vi "S8300E_ENT_TEST_MODE_DVT.vi"() -> ()   [LabVIEW 2011]
panel:
  out "Found login?":bool
  out "TELNET-KEYWORD2-AfterLogin":string
  out "TELNET-KEYWORD1-AfterLogin":string
  out "TELNET-PATH":string
  out "TELNET-PASSWORD":string
  out "TELNET-ID":string
  out "Debug View":string
  out "cmd-list":T1(array[cluster])
  out "cmd":string
  out "VISA resource name out":refnum<visa-resource-name>
  out "進行狀況":string
  out "BEGIN TIME":u32
  # "Error Code:MB-NG"
  # "S8300E Enter Test Mode"
  # "2015-1-26"
  # "COM9 115200"
  # "1.本程式不會給UUT 上電,需先執行上電程式\n2.在執行本程式前,需先執行上電程式(S8300E_BootupTime_Delay)\n3.本程式只是給UUT ROOT權限 與 切換到測試程式路徑"
  # "Write Command :Char by Char"
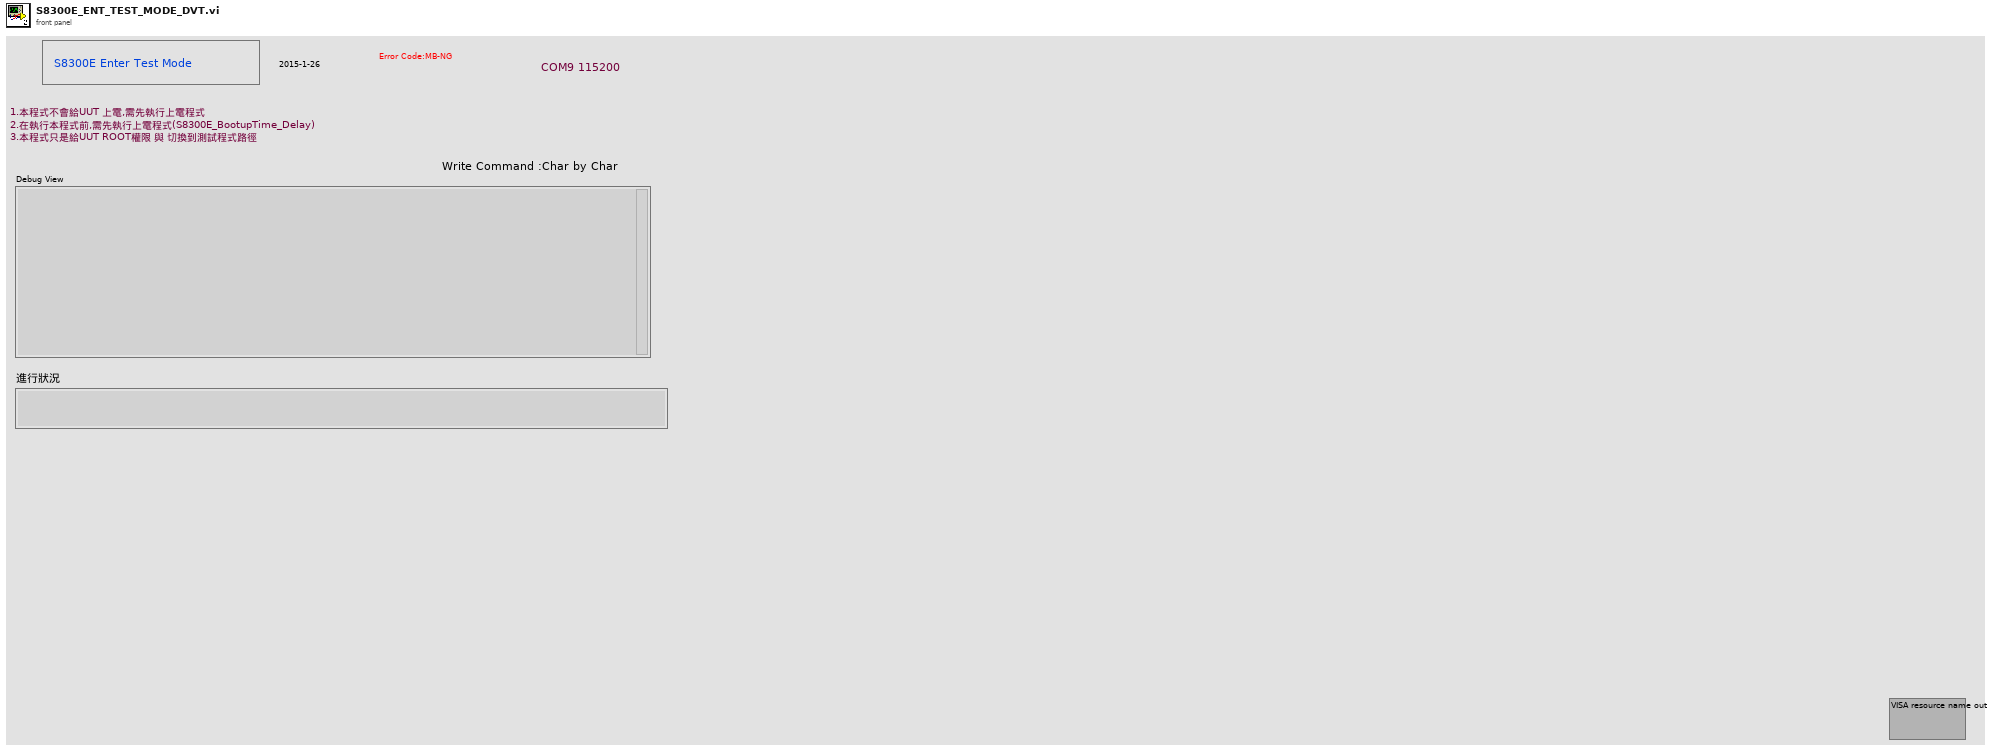
[diagram p1: front panel]
types:
  T1 = cluster{string, "Find this String":string, "Status":string}[]
  T2 = cluster{string, "TELNET-KEYWORD1-AfterLogin":string, "Status":string}
  T3 = cluster{string, "Search String":string, "Status":string}
  T4 = cluster{string, "TELNET-KEYWORD2-AfterLogin":string, "Status":string}
  T5 = cluster{string, "TELNET-KEYWORD2-AfterLogin":string, "Status":string}[]
  T6 = cluster{string, "Find this String":string, "Status":string}
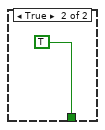
[diagram p4: hidden frame]
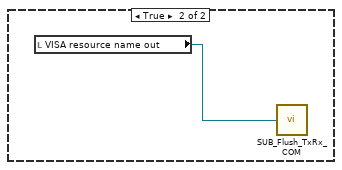
[diagram p5: hidden frame]
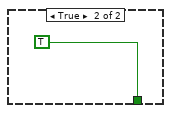
[diagram p7: hidden frame]
diagram:
  n1 = flat-sequence {
    tunnel: [w38] -> w2
    tunnel: w2 -> [w39]
    tunnel: [w144] -> w1
    tunnel: w1 -> [w150]
    frame #0 {
      n2 = Tick Count (ms)() -> (millisecond timer value=→"BEGIN TIME":u32)
    }
    frame #1 {
      n3 = call "SUB_COM1_CLOSE.vi"("VISA resource name"=refnum<visa-resource-name> "COM9") -> ()  [unwired: 3 in]
      n4 = property on="進行狀況" class="Str"("Blinking"=TRUE) -> ()  [unwired: 2 in, 2 out]
      "進行狀況" <- "進入測試準備中...." ("進行狀況")
      "Debug View" <- ""
    }
    frame #2 {
      n5 = call "SUB_COM9_INIT.vi"("baud rate"=u32 115200) -> ("VISA resource name out"=→"VISA resource name out":refnum<visa-resource-name>)  [unwired: 1 in, 1 out]
    }
    frame #3 {
      n6 = call "SUB_ReadScript_File.vi"("Script FileName"="S8300E_sfcs_misc.txt" ("Search Filename in Folder")) -> ("text"=w18:string)  [unwired: 1 in, 2 out]
      n7 = call "SUB_FindSpecificString.vi"("Find this String"="TELNET_PASSWORD=", "String data"=w18) -> ("before \"; \" string"=w24:string, "Found"=w31:bool)  [unwired: 2 in]
      n8 = call "SUB_FindSpecificString.vi"("Find this String"="TELNET_PATH=", "String data"=w18) -> ("before \"; \" string"=w22:string, "Found"=w29:bool)  [unwired: 2 in]
      n9 = call "SUB_FindSpecificString.vi"("Find this String"="TELNET_ID=", "String data"=w18) -> ("before \"; \" string"=w26:string, "Found"=w32:bool)  [unwired: 2 in]
      n10 = To Lower Case(string=w26) -> (all lower case string=→"TELNET-ID":string)
      n11 = To Lower Case(string=w24) -> (all lower case string=→"TELNET-PASSWORD":string)
      n12 = To Lower Case(string=w22) -> (all lower case string=→"TELNET-PATH":string)
      n13 = call "SUB_FindSpecificString.vi"("Find this String"="TELNET_KEYWORD1_AFTERLOG_IN=", "String data"=w18) -> ("before \"; \" string"=w20:string, "Found"=w14:bool)  [unwired: 2 in]
      n14 = call "SUB_FindSpecificString.vi"("Find this String"="TELNET_KEYWORD2_AFTERLOG_IN=", "String data"=w18) -> ("before \"; \" string"=w16:string, "Found"=w13:bool)  [unwired: 2 in]
      n15 = To Lower Case(string=w20) -> (all lower case string=→"TELNET-KEYWORD1-AfterLogin":string)
      n16 = To Lower Case(string=w16) -> (all lower case string=→"TELNET-KEYWORD2-AfterLogin":string)
      n17 = And(x=w32, y=w31) -> (x .and. y?=w30:bool)
      n18 = And(x=w30, y=w29) -> (x .and. y?=w12:bool)
      n19 = And(x=w14, y=w13) -> (x .and. y?=w11:bool)
      n20 = And(x=w12, y=w11) -> (x .and. y?=w10:bool)
      n21 = case shown="False" w10 {
        frame False {
          n22 = flat-sequence {
            frame #0 {
              n23 = call "Display Message to User"() -> ()  [unwired: 10 in, 2 out]
            }
            frame #1 {
              n24 = call "SUB_Writelog.vi"("Pass/Fail"="Fail:S8300E_ENT_TEST_MODE_NEW") -> ()  [unwired: 2 in]
            }
            frame #2 {
              n25 = Quit LabVIEW(quit? (T)=TRUE) -> ()
            }
          }
        }
        frame True {
        }
      }
    }
    frame #4 {
      n26 = Tick Count (ms)() -> (millisecond timer value=w38:u32)
    }
    frame #5 {
      n27 = while {
        tunnel: w39 -> [w43]
        stop <- w47 stop-if-true
        w41 = "\r"
        n28 = local read "VISA resource name out"() -> (w54:refnum<visa-resource-name>)
        n29 = Concatenate Strings(w41, w41) -> (w40:string)
        n30 = call "SUB_COM1Wrt.vi"("VISA resource name"=w54, "write buffer"=w40) -> ("duplicate VISA resource name"=w56:refnum<visa-resource-name>)  [unwired: 1 in, 1 out]
        n31 = Tick Count (ms)() -> (millisecond timer value=w53:u32)
        n32 = Subtract(x=w53, y=w43) -> (x-y=w52:u32)
        n33 = call "SUB_ContinueCom1Read.vi"("Numeric"=200, "duplicate VISA resource name 2"=w56) -> ("String"=w45:string)  [unwired: 1 in, 2 out]
        n34 = Divide(x=w52, y=u32 1000) -> (x/y=w50:dbl)
        n35 = Wait (ms)(milliseconds to wait=u32 150) -> ()  [unwired: 1 out]
        n36 = Greater?(x=w50, y=u32 20) -> (0:w48:bool)
        n37 = call "SUB_FindSpecificString.vi"("Find this String"="s8300e login:", "String data"=w45) -> ("Found"=w46:bool)  [unwired: 2 in, 1 out]
        "Found login?" <- w46
        n38 = Or(x=w46, y=w48) -> (x .or. y?=w47:bool)
        n39 = local write "Debug View"(w45) -> ()
      }
    }
    frame #6 {
      n40 = local write "Found login?"(FALSE ("Found login?")) -> ()
    }
    frame #7 {
      n41 = local read "Found login?"() -> (w58:bool)
      n42 = case shown="False" w58 {
        frame False {
          n43 = while {
            stop <- w61 stop-if-true
            n44 = local read "VISA resource name out"() -> (w66:refnum<visa-resource-name>)
            n45 = Tick Count (ms)() -> (millisecond timer value=w65:u32)
            n46 = call "SUB_WR_COM1_CbyCFindString_timeout.vi"("Begin time"=w65, "Find this String"="s8300e login:", "Timeout Seccond"=5.0, "cmd string"="\r", "duplicate VISA resource name 2"=w66) -> ("Output String"=w60:string, "Found String"=w62:bool)  [unwired: 2 out]
            n47 = local write "Debug View"(w60) -> ()
            n48 = case shown="False" w62 {
              tunnel: w60 -> [w67 _]
              tunnel: [_ TRUE] -> w61
              frame False {
                n49 = call "SUB_YESNO.vi"("Debug View"=w67, "Status"="UUT 未開機完成Ready") -> ("yes/no"=w70:enum32{"No Selection", "Yes", "No", "None"})  [unwired: 1 in]
                n50 = Equal?(x=w70, y=enum32{"No Selection", "Yes", "No", "None"}."No") -> (x = y?=w68:bool)
                n51 = case shown="True" w68 {
                  frame False {
                  }
                  frame True {
                    n52 = flat-sequence {
                      frame #0 {
                        n53 = call "SUB_COM1_CLOSE.vi"("VISA resource name"=refnum<visa-resource-name> "COM9") -> ()  [unwired: 3 in]
                      }
                      frame #1 {
                        n54 = call "SUB_Writelog.vi"("Pass/Fail"="Fail:S8300E_ENT_TEST_MODE_NEW") -> ()  [unwired: 2 in]
                      }
                      frame #2 {
                        n55 = call "SUB_SFCS_SendResult.vi"("ErrorCode"="MB-NG", "PASS_Fail (1/0)"=i8 0) -> ()  [unwired: 1 out]
                      }
                      frame #3 {
                        n56 = Quit LabVIEW(quit? (T)=TRUE) -> ()
                      }
                    }
                  }
                }
              }
              frame True {
              }
            }
          }
        }
        frame True {
          n57 = local read "VISA resource name out"() -> (w78:refnum<visa-resource-name>)
          n58 = call "SUB_Flush_TxRx_COM.vi"("VISA resource name"=w78) -> ()  [unwired: 1 in]
        }
      }
    }
    frame #8 {
      w92 = "change to specific directory"  # Status
      w95 = "Login root Password"  # Status
      w96 = "root@"  # Search String
      w99 = "Switch to root privilege"  # Status
      w100 = "password for s8300e:"  # Search String
      w104 = "Login  Password"  # Status
      w107 = "Login Account"  # Status
      w108 = "Password:"  # Search String
      n59 = local read "TELNET-PASSWORD"() -> (w84:string)
      n60 = local read "TELNET-PASSWORD"() -> (w82:string)
      n61 = local read "TELNET-KEYWORD1-AfterLogin"() -> (w83:string)
      n62 = local read "TELNET-KEYWORD2-AfterLogin"() -> (w80:string)
      n63 = local read "TELNET-PATH"() -> (w81:string)
      n64 = local read "TELNET-ID"() -> (w85:string)
      n65 = Concatenate Strings(w84, "\r") -> (w105:string)
      n66 = Concatenate Strings(w85, "\r") -> (w109:string)
      "cmd" <- w109
      n67 = Concatenate Strings("sudo -i" ("string"), "\r") -> (w101:string)
      n68 = Concatenate Strings(w82, "\r") -> (w97:string)
      n69 = Concatenate Strings("cd  /", w81, "\r") -> (w93:string)
      n70 = Bundle(w105, "TELNET-KEYWORD1-AfterLogin"=w83, "Status"=w104) -> (w90:T2)  [unwired: 1 in]
      n71 = Bundle(w109, "Search String"=w108, "Status"=w107) -> (w91:T3)  [unwired: 1 in]
      n72 = Bundle(w101, "Search String"=w100, "Status"=w99) -> (w89:T3)  [unwired: 1 in]
      n73 = Bundle(w97, "Search String"=w96, "Status"=w95) -> (w88:T3)  [unwired: 1 in]
      n74 = Bundle(w93, "TELNET-KEYWORD2-AfterLogin"=w80, "Status"=w92) -> (w87:T4)  [unwired: 1 in]
      n75 = Build Array(w91, w90, w89, w88, w87) -> (→"cmd-list":T5)
    }
    frame #9 {
      n76 = call "SUB_ContinueCom1Read.vi"("Numeric"=2500, "duplicate VISA resource name 2"=refnum<visa-resource-name> "COM9") -> ("duplicate VISA resource name"=w112:refnum<visa-resource-name>)  [unwired: 1 in, 2 out]
      n77 = call "SUB_Flush_TxRx_COM.vi"("VISA resource name"=w112) -> ()  [unwired: 1 in]
    }
    frame #10 {
      n78 = local read "cmd-list"() -> (w115:T1)
      n79 = Array Size(array=w115) -> (size(s)=w114:i32)
      n80 = for {
        N: w114 -> [_]
        i -> [w116]
        n81 = while {
          tunnel: w116 -> [w128]
          stop <- w127 stop-if-true
          n82 = local read "cmd-list"() -> (w126:T1)
          n83 = local read "VISA resource name out"() -> (w122:refnum<visa-resource-name>)
          n84 = Tick Count (ms)() -> (millisecond timer value=w121:u32)
          n85 = Index Array(array=w126, index=w128) -> (element=w125:T6)
          n86 = Unbundle(w125) -> (w123:string, "Find this String"=w118:string, "Status"=w124:string)
          n87 = call "SUB_WR_COM1_CbyCFindString_timeout.vi"("Begin time"=w121, "Find this String"=w118, "Timeout Seccond"=5.0, "cmd string"=w123, "duplicate VISA resource name 2"=w122) -> ("Output String"=w117:string, "Found String"=w119:bool)  [unwired: 2 out]
          n88 = local write "進行狀況"(w124) -> ()
          n89 = case shown="False" w119 {
            tunnel: [_ TRUE] -> w127
            tunnel: w117 -> [w129 _]
            frame False {
              n90 = local read "進行狀況"() -> (w131:string)
              n91 = Concatenate Strings("失敗!" ("string"), w131) -> (w130:string)
              n92 = call "SUB_YESNO.vi"("Debug View"=w129, "Status"=w130) -> ("yes/no"=w135:enum32{"No Selection", "Yes", "No", "None"})  [unwired: 1 in]
              n93 = Equal?(x=w135, y=enum32{"No Selection", "Yes", "No", "None"}."No") -> (x = y?=w133:bool)
              n94 = case shown="True" w133 {
                frame False {
                }
                frame True {
                  n95 = flat-sequence {
                    frame #0 {
                      n96 = call "SUB_COM1_CLOSE.vi"("VISA resource name"=refnum<visa-resource-name> "COM9") -> ()  [unwired: 3 in]
                    }
                    frame #1 {
                      n97 = call "SUB_Writelog.vi"("Pass/Fail"="Fail:S8300E_ENT_TEST_MODE_NEW") -> ()  [unwired: 2 in]
                    }
                    frame #2 {
                      n98 = call "SUB_SFCS_SendResult.vi"("ErrorCode"="MB-NG", "PASS_Fail (1/0)"=i8 0) -> ()  [unwired: 1 out]
                    }
                    frame #3 {
                      n99 = Quit LabVIEW(quit? (T)=TRUE) -> ()
                    }
                  }
                }
              }
            }
            frame True {
            }
          }
        }
      }
    }
    frame #11 {
      n100 = local read "VISA resource name out"() -> (w146:refnum<visa-resource-name>)
      n101 = call "SUB_COM1Wrt.vi"("VISA resource name"=w146, "write buffer"="\r") -> ("duplicate VISA resource name"=w147:refnum<visa-resource-name>)  [unwired: 1 in, 1 out]
      n102 = call "SUB_ContinueCom1Read.vi"("Numeric"=200, "duplicate VISA resource name 2"=w147) -> ("String"=w144:string, "duplicate VISA resource name"=w145:refnum<visa-resource-name>)  [unwired: 1 in, 1 out]
      n103 = call "SUB_COM1_CLOSE.vi"("VISA resource name"=w145) -> ()  [unwired: 3 in]
    }
    frame #12 {
      w149 = "\r"
      n104 = Tick Count (ms)() -> (millisecond timer value=w153:u32)
      n105 = local read "BEGIN TIME"() -> (w154:u32)
      n106 = call "SUB_CAL_TESTTIME.vi"("Test Item name"="S8300E_ENT_TEST_MODE_NEW", "Stop tick time"=w153, "Start tick time"=w154) -> ("Test Time output"=w148:string)  [unwired: 2 in]
      n107 = Concatenate Strings("Pass:S8300E_ENT_TEST_MODE_NEW" ("string"), w149, w150, w149, w148) -> (w151:string)
      n108 = call "SUB_Writelog.vi"("Pass/Fail"=w151) -> ()  [unwired: 2 in]
    }
    frame #13 {
      n109 = call "SUB_Flush_TxRx_COM.vi"("VISA resource name"=refnum<visa-resource-name> "COM9") -> ()  [unwired: 1 in]
    }
    frame #14 {
      n110 = call "SUB_COM1_CLOSE.vi"("VISA resource name"=refnum<visa-resource-name> "COM9") -> ()  [unwired: 3 in]
    }
    frame #15 {
      n111 = Quit LabVIEW(quit? (T)=TRUE) -> ()
    }
  }
